vi "Numeric Representation.vi"(8 "error in (no error)":errorcluster, 10 "Representation":T1, 11 "GObject in":refnum<vi>) -> (0 "error out":errorcluster, 2 "is numeric?":bool, 3 "GObject out":refnum<vi>)   [LabVIEW 2019, in "Builtins.lvlib"]
doc: "Changes the numeric representation on the selected front panel or block diagram objects. Constant labels are updated the abreviated numeric type (i.e. \"U8\", \"I32\", etc.).\n\nCreated by: Ryan Pacini"
uses:
  Builtins.lvlib
  <vilib>/numeric/LVNumericRepresentation.ctl
  Label Position.ctl
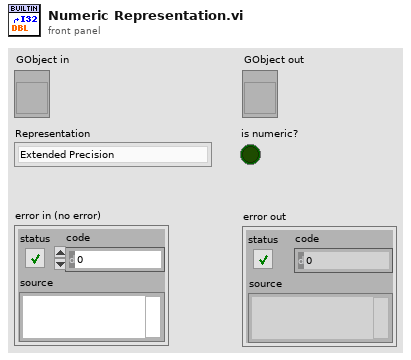
[diagram p1: front panel]
types:
  T1 = typedef "LVNumericRepresentation.ctl" = enum32{"Extended Precision", "Double Precision", "Single Precision", "Long", "Word", "Byte", "Unsigned Long", "Unsigned Word", "Unsigned Byte", "Complex Extended", "Complex Double", "Complex Single", "Quad", "Unsigned Quad", "Fixed-Point"}
  T2 = typedef "Builtins.lvlib/Label Position.ctl" = enum8{"Unchanged", "Top-left", "Top-middle", "Top-right", "Right-top", "Right-middle", "Right-bottom", "Bottom-right", "Bottom-middle", "Bottom-left", "Left-bottom", "Left-middle", "Left-top"}
  T3 = typedef "LVRectTypeDef.ctl" = cluster{"Left":i16, "Top":i16, "Right":i16, "Bottom":i16}
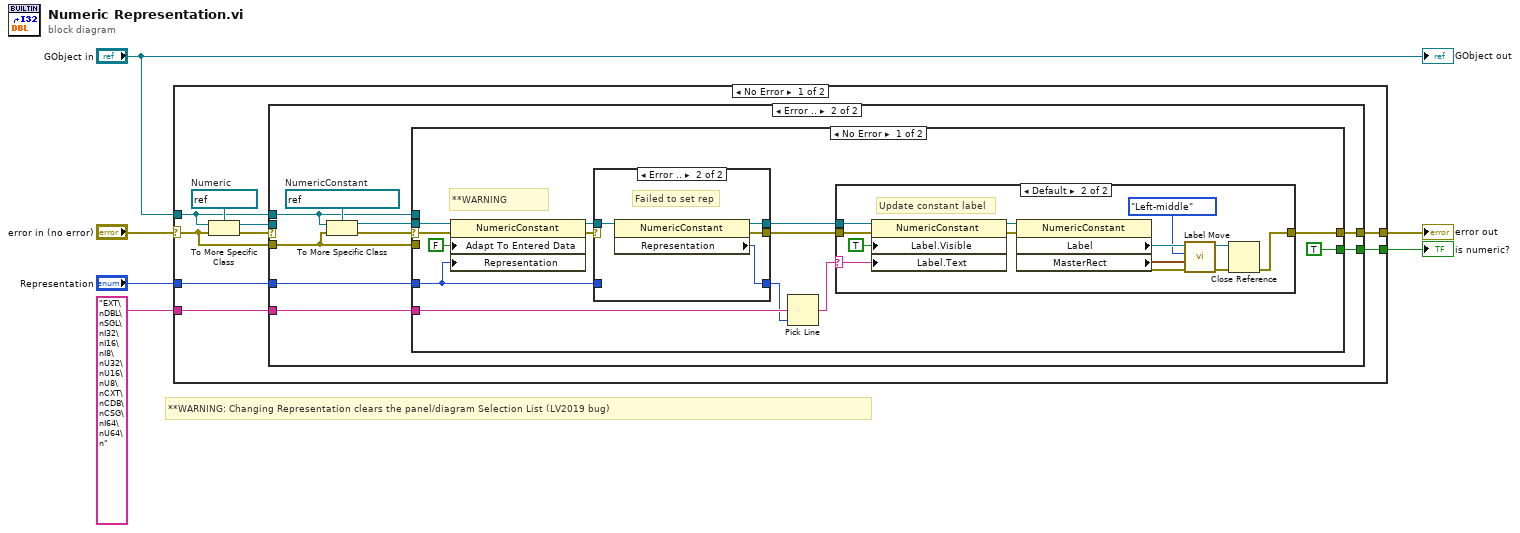
[diagram p0: block diagram]
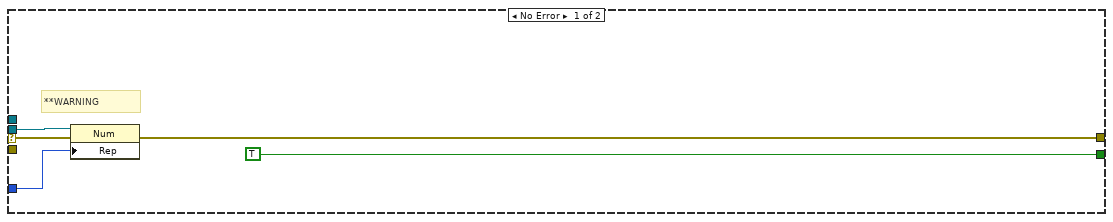
[diagram p2: hidden frame]
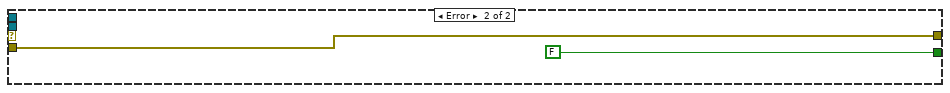
[diagram p5: hidden frame]
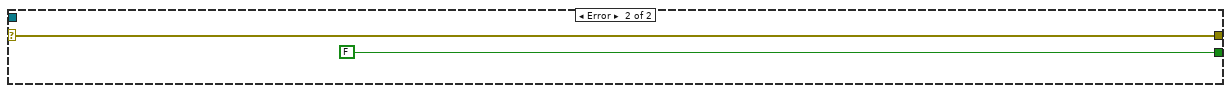
[diagram p6: hidden frame]
diagram:
  # "**WARNING: Changing Representation clears the panel/diagram Selection List (LV2019 bug)"
  n1 = case shown="No Error" "error in (no error)" {
    selector: "error in (no error)" -> [w11 w67]
    tunnel: "GObject in" -> [w13 _]
    tunnel: "Representation" -> [w8 _]
    tunnel: [w15 w67] -> w3
    tunnel: [w9 FALSE] -> w2
    tunnel: "EXT\nDBL\nSGL\nI32\nI16\nI8\nU32\nU16\nU8\nCXT\nCDB\nCSG\nI64\nU64\n" -> [w7 _]
    frame No Error {
      w14 = refnum<vi> refnum  # Numeric
      n2 = To More Specific Class(target class=w14, reference=w13, error in=w11) -> (specific class reference=w10:refnum<vi>, error out=w12:errorcluster)
      n3 = case shown="Error .." w12 {
        selector: w12 -> [w20 _]
        tunnel: w8 -> [w18 w26]
        tunnel: [w17 w25] -> w15
        tunnel: w13 -> [_ w24]
        tunnel: w11 -> [_ w23]
        tunnel: w10 -> [w19 _]
        tunnel: [TRUE w22] -> w9
        tunnel: w7 -> [_ w21]
        frame No Error {
          # "**WARNING"
          n4 = property class="Num"(reference=w19, error in=w20, "Rep"=w18) -> (error out=w17:errorcluster)  [unwired: 1 out]
        }
        frame Error {
          w29 = refnum<vi> refnum  # NumericConstant
          n5 = To More Specific Class(target class=w29, reference=w24, error in=w23) -> (specific class reference=w28:refnum<vi>, error out=w27:errorcluster)
          n6 = case shown="No Error" w27 {
            selector: w27 -> [w42 _]
            tunnel: w28 -> [w41 _]
            tunnel: w26 -> [w31 _]
            tunnel: [w38 w65] -> w25
            tunnel: w24 -> [_ _]
            tunnel: w23 -> [_ w65]
            tunnel: [TRUE FALSE] -> w22
            tunnel: w21 -> [w37 _]
            frame No Error {
              # "**WARNING"
              n7 = property class="NumericConstant"(reference=w41, error in=w42, "Adapt To Entered Data"=FALSE, "Representation"=w31) -> (reference out=w34:refnum<vi>, error out=w39:errorcluster)
              n8 = case shown="Error .." w39 {
                selector: w39 -> [w43 _]
                tunnel: [w43 w49] -> w35
                tunnel: w34 -> [w44 w48]
                tunnel: [w44 w47] -> w33
                tunnel: [w45 w46] -> w32
                tunnel: w31 -> [w45 _]
                frame No Error {
                }
                frame Error {
                  # "Failed to set rep"
                  n9 = property class="NumericConstant"(reference=w48) -> (reference out=w47:refnum<vi>, error out=w49:errorcluster, "Representation"=w46:T1)  [unwired: 1 in]
                }
              }
              n10 = Pick Line(multi-line string=w37, line index=w32) -> (output string=w36:string)  [unwired: 1 in]
              n11 = case shown="Default" w36 {
                selector: w36 -> [_ w60]
                tunnel: w35 -> [w50 w63]
                tunnel: [w50 w53] -> w38
                tunnel: w33 -> [_ w62]
                frame "" {
                }
                frame Default {
                  # "Update constant label"
                  n12 = property class="NumericConstant"(reference=w62, error in=w63, "Label.Visible"=TRUE, "Label.Text"=w60) -> (reference out=w58:refnum<vi>, error out=w59:errorcluster)
                  n13 = property class="NumericConstant"(reference=w58, error in=w59) -> (error out=w52:errorcluster, "Label"=w57:refnum<vi>, "MasterRect"=w56:T3)  [unwired: 1 out]
                  n14 = call "Label Move.vi"("error in (no error)"=w52, "Owner Master Bounds Rect"=w56, "Label Position"=Label_Position."Left-middle", "Label in"=w57) -> ("error out"=w54:errorcluster, "dup Label"=w55:refnum<vi>)  [unwired: 6 in]
                  n15 = Close Reference(reference=w55, error in (no error)=w54) -> (error out=w53:errorcluster)
                }
              }
            }
            frame Error {
            }
          }
        }
      }
    }
    frame Error {
    }
  }
  "error out" <- w3
  "is numeric?" <- w2
  "GObject out" <- "GObject in"
